vi "niRFUtil MT UTIL GF2 Primative Poly LUT.vi"() -> (0 "GF(2) Primative Polynomials":u32[](array[numeric]))   [LabVIEW 2015, in "niRFUtil.lvlib"]
uses:
  niRFUtil.lvlib
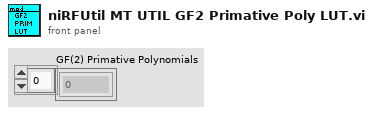
[diagram p1: front panel]
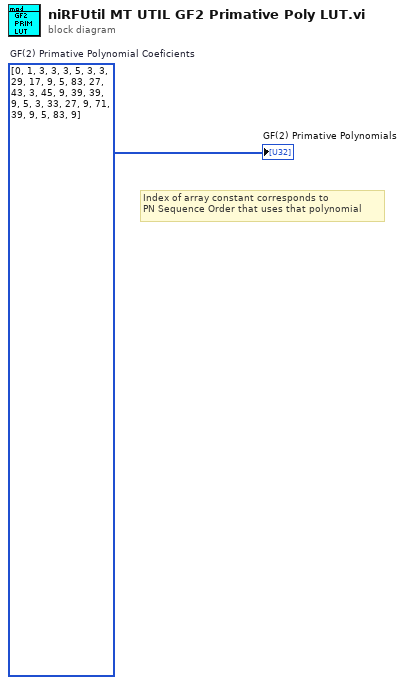
[diagram p0: block diagram]
diagram:
  w1 = u32[] [0, 1, 3, 3, 3, 5, 3, 3, 29, 17, 9, 5, 83, 27, 43, 3, 45, 9, 39, 39, 9, 5, 3, 33, 27, 9, 71, 39, 9, 5, 83, 9]  # GF(2) Primative Polynomial Coeficients
  # "Index of array constant corresponds to\nPN Sequence Order that uses that polynomial"
  "GF(2) Primative Polynomials" <- w1
